vi "虚拟放射源设置-beta吸收.vi"(0 "计数率":u32=20 max=2000000, 1 "仪器使能":i32 max=1, 2 "衰减系数":dbl=1.0 min=0.0 max=1.0) -> ()   [LabVIEW 2014]
panel:
  in  "最小时间间隔":u16=20 min=15 step=1
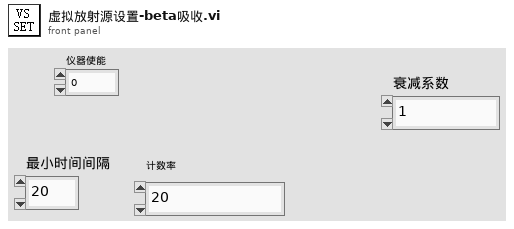
[diagram p1: front panel]
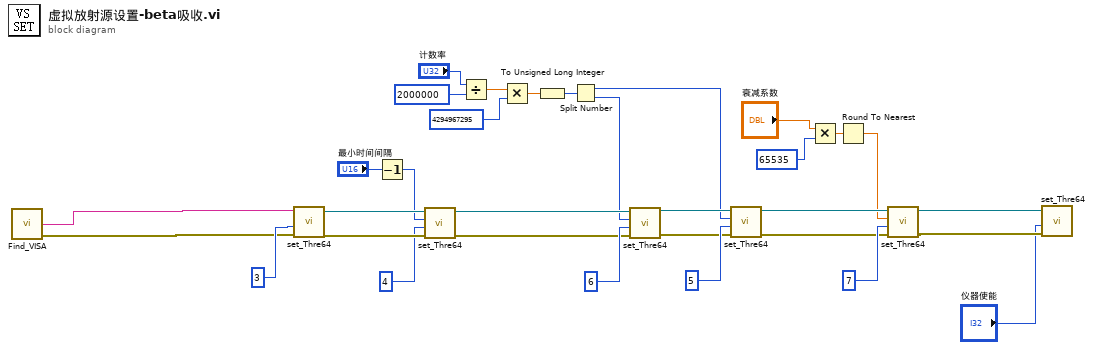
[diagram p0: block diagram]
diagram:
  n1 = call "Find_VISA.vi"() -> ("错误输出"=w3:errorcluster, "虚拟放射源VISA"=w2:string)  [unwired: 3 in, 1 out]
  n2 = call "set_Thre64.vi"("错误输入（无错误）"=w3, "命令"=3, "VISA资源名称"=w2) -> ("错误输出"=w31:errorcluster, "VISA资源名称输出"=w32:refnum<visa-resource-name>)  [unwired: 7 in]
  n3 = Decrement(x="最小时间间隔") -> (x-1=w27:u16)
  n4 = call "set_Thre64.vi"("错误输入（无错误）"=w31, "命令"=4, "数字"=w27, "VISA资源名称"=w32) -> ("错误输出"=w25:errorcluster, "VISA资源名称输出"=w26:refnum<visa-resource-name>)  [unwired: 6 in]
  n5 = Divide(x="计数率", y=u32 2000000) -> (x/y=w22:dbl)
  n6 = Multiply(x=w22, y=u32 4294967295) -> (x*y=w17:dbl)
  n7 = To Unsigned Long Integer(number=w17) -> (unsigned 32bit integer=w16:u32)
  n8 = Split Number(x=w16) -> (hi(x)=w14:u16, lo(x)=w15:u16)
  n9 = call "set_Thre64.vi"("错误输入（无错误）"=w25, "命令"=6, "数字"=w15, "VISA资源名称"=w26) -> ("错误输出"=w18:errorcluster, "VISA资源名称输出"=w19:refnum<visa-resource-name>)  [unwired: 6 in]
  n10 = call "set_Thre64.vi"("错误输入（无错误）"=w18, "命令"=5, "数字"=w14, "VISA资源名称"=w19) -> ("错误输出"=w11:errorcluster, "VISA资源名称输出"=w12:refnum<visa-resource-name>)  [unwired: 6 in]
  n11 = Multiply(x="衰减系数", y=u32 65535) -> (x*y=w8:dbl)
  n12 = Round To Nearest(number=w8) -> (nearest integer value=w7:dbl)
  n13 = call "set_Thre64.vi"("错误输入（无错误）"=w11, "命令"=7, "数字"=w7, "VISA资源名称"=w12) -> ("错误输出"=w5:errorcluster, "VISA资源名称输出"=w4:refnum<visa-resource-name>)  [unwired: 6 in]
  n14 = call "set_Thre64.vi"("错误输入（无错误）"=w5, "命令"="仪器使能", "VISA资源名称"=w4) -> ()  [unwired: 7 in, 2 out]
